vi "Test Math.vi"(8 "error in (no error)":errorcluster) -> (0 "error out":errorcluster)   [LabVIEW 2020]
uses:
  d5c845a2-4865-4f6a-83f0-4ce0aaa7851f.vi
  f8819591-6fbe-434b-b3d2-538ddc5f099c.vi
  626d8354-143d-466b-b830-8d7a47135a8c.vi
  0a54e210-7b74-4968-9a19-3f53a999a716.vi
  aa93a00a-f4f6-4502-85dd-738e6c144677.vi
  fa01e91c-d5a3-4e85-992f-aaeb5359cc34.vi
  4f3af36e-3c59-4f7f-82ad-0b3053415c44.vi/6238254b-de7a-41d2-bc88-34d202be72c0.vi
  4f3af36e-3c59-4f7f-82ad-0b3053415c44.vi/541a0482-0882-4cce-b454-9f4ea1bdb34c.vi
  f8819591-6fbe-434b-b3d2-538ddc5f099c.vi/6238254b-de7a-41d2-bc88-34d202be72c0.vi
  f8819591-6fbe-434b-b3d2-538ddc5f099c.vi/16b9c82e-e8e3-4cdd-b95c-cb8e07aaddae.vi
  f8819591-6fbe-434b-b3d2-538ddc5f099c.vi/bfe79359-bfac-4602-94ca-4042fcd6f890.vi
  626d8354-143d-466b-b830-8d7a47135a8c.vi/6238254b-de7a-41d2-bc88-34d202be72c0.vi
  626d8354-143d-466b-b830-8d7a47135a8c.vi/16b9c82e-e8e3-4cdd-b95c-cb8e07aaddae.vi
  626d8354-143d-466b-b830-8d7a47135a8c.vi/bfe79359-bfac-4602-94ca-4042fcd6f890.vi
  0a54e210-7b74-4968-9a19-3f53a999a716.vi/6238254b-de7a-41d2-bc88-34d202be72c0.vi
  0a54e210-7b74-4968-9a19-3f53a999a716.vi/bfe79359-bfac-4602-94ca-4042fcd6f890.vi
  <vilib>/addons/_JKI Toolkits/Caraya/classes/Assert/Assert Equal Value and Type_Variant.vi
  <vilib>/addons/_JKI Toolkits/Caraya/classes/Test/Test.lvclass
  <vilib>/addons/_JKI Toolkits/Caraya/classes/Assert/Assert.lvclass
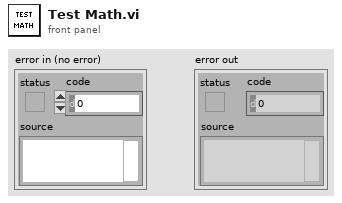
[diagram p1: front panel]
types:
  T1 = cluster{"Value":i32, "Start":i32, "Length":i32}[]
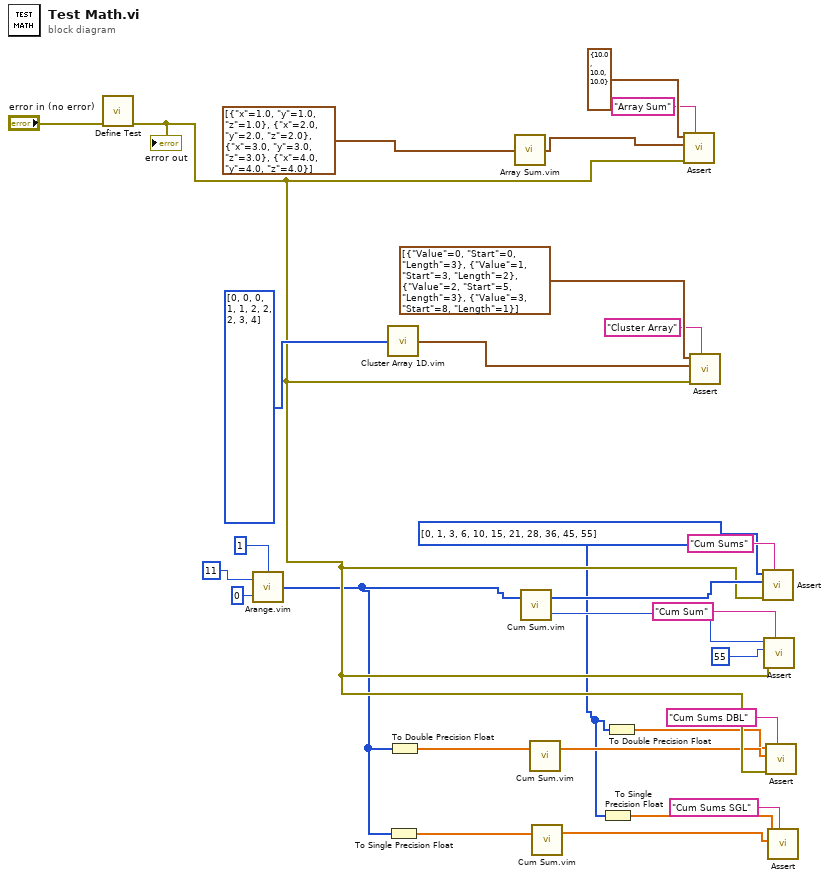
[diagram p0: block diagram]
diagram:
  w2 = i32[] [0, 1, 3, 6, 10, 15, 21, 28, 36, 45, 55] ("Cumulated Products Out")
  n1 = call <vilib>:"Define Test.vi"("error in (no error)"="error in (no error)") -> ("error out"=w10:errorcluster)  [unwired: 10 in]
  "error out" <- w10
  n2 = call "Arange.vim"("Step"=1, "Low (Incl, type)"=0, "High (Excl)"=11) -> ("Array"=w6:i32[])
  n3 = call "Cluster Array 1D.vim"("Array"=i32[] [0, 0, 0, 1, 1, 2, 2, 2, 3, 4]) -> ("Clusters"=w22:T1)
  n4 = To Single Precision Float(number=w6) -> (single precision float=w5:sgl[])
  n5 = To Double Precision Float(number=w6) -> (double precision float=w11:dbl[])
  n6 = call "Array Sum.vim"("Array"=cluster{"x":dbl, "y":dbl, "z":dbl}[] [{"x"=1.0, "y"=1.0, "z"=1.0}, {"x"=2.0, "y"=2.0, "z"=2.0}, {"x"=3.0, "y"=3.0, "z"=3.0}, {"x"=4.0, "y"=4.0, "z"=4.0}]) -> ("Sum"=w27:cluster{"x":dbl, "y":dbl, "z":dbl})
  n7 = call "Cum Sum.vim"("Array In"=w6) -> ("Cumulated Sum"=w13:i64, "Cumulated Sums Out"=w15:i32[])  [unwired: 1 in]
  n8 = call "Cum Sum.vim"("Array In"=w11) -> ("Cumulated Sums Out"=w9:dbl[])  [unwired: 1 in, 1 out]
  n9 = call "Cum Sum.vim"("Array In"=w5) -> ("Cumulated Sums Out"=w4:sgl[])  [unwired: 1 in, 1 out]
  n10 = To Single Precision Float(number=w2) -> (single precision float=w3:sgl[])
  n11 = To Double Precision Float(number=w2) -> (double precision float=w8:dbl[])
  n12 = call-poly <vilib>:"Assert.vi"("Label"="Array Sum", "error in (no error)"=w10, "Y"=w27, "X"=cluster{"x":dbl, "y":dbl, "z":dbl} {"x"=10.0, "y"=10.0, "z"=10.0} ("Sum")) -> ()  [unwired: 7 in, 1 out]
  n13 = call-poly <vilib>:"Assert.vi"("Label"="Cluster Array", "error in (no error)"=w10, "Y"=w22, "X"=T1 [{"Value"=0, "Start"=0, "Length"=3}, {"Value"=1, "Start"=3, "Length"=2}, {"Value"=2, "Start"=5, "Length"=3}, {"Value"=3, "Start"=8, "Length"=1}] ("Clusters")) -> ()  [unwired: 7 in, 1 out]
  n14 = call-poly <vilib>:"Assert.vi"("Label"="Cum Sums", "error in (no error)"=w10, "Y"=w15, "X"=w2) -> ()  [unwired: 7 in, 1 out]
  n15 = call-poly <vilib>:"Assert.vi"("Label"="Cum Sum", "error in (no error)"=w10, "Y"=i64 55 ("Cumulated Sum"), "X"=w13) -> ()  [unwired: 7 in, 1 out]
  n16 = call-poly <vilib>:"Assert.vi"("Label"="Cum Sums DBL", "error in (no error)"=w10, "Y"=w9, "X"=w8) -> ()  [unwired: 7 in, 1 out]
  n17 = call-poly <vilib>:"Assert.vi"("Label"="Cum Sums SGL", "Y"=w4, "X"=w3) -> ()  [unwired: 8 in, 1 out]
